vi "LilyPad_RB.vi"() -> ()   [LabVIEW 2012]
uses:
  <userlib>/BotSpeak/VIs/Direct/BotSpeak_Control.ctl
panel:
  in  "Bot Settings":T1
  out "List":string[](array[string])
  out "page":u8
  in  "Intro Help":bool
  in  "Previous":bool
  in  "Next":bool
  in  "Stop Button":bool
  in  "Pages":T2(tab)
  in  "Test Button":bool
  in  "Com Port":u16(ring)
  in  "Hardware":u16(ring) items=["Arduino Uno", "BeagleBone Serial", "BeagleBone", "Console Only", "EV3", "EvalRIO", "Launchpad", "PICAXE 80M", "Raspberry Pi", "Thymio"]
  out "firmware":dbl
  in  "Open":bool
  in  "Port":u8=13
  in  "State":enum16{"LO", "HI"}(ring)
  in  "Run":bool
  # "Getting Started\n\nThe goal of this book is to get you started in LabVIEW with the Lilypad - you will need 1 lilypad - please connect it up."
  # "Test BotSpeak\n\nThe next step is to test it out.  Choose your hardware and port (if you have not plugged your LilyPad in yet, plug it in and select Arduino Uno).  Push TEST to text the connection and see if you get Firmware 0.9 back."
  # "Test LilyPad\n\nPush the Run button - does the light go off?  Change it from LO to HI - and run it again.  What happens? Try changing the Port - from pin 13 to some other number.  This is called a LabVIEW diagram - it is where your program resides - this program is simple - it changes the state of pin 13.  Click on the Open button to open a slightly more complicated program."
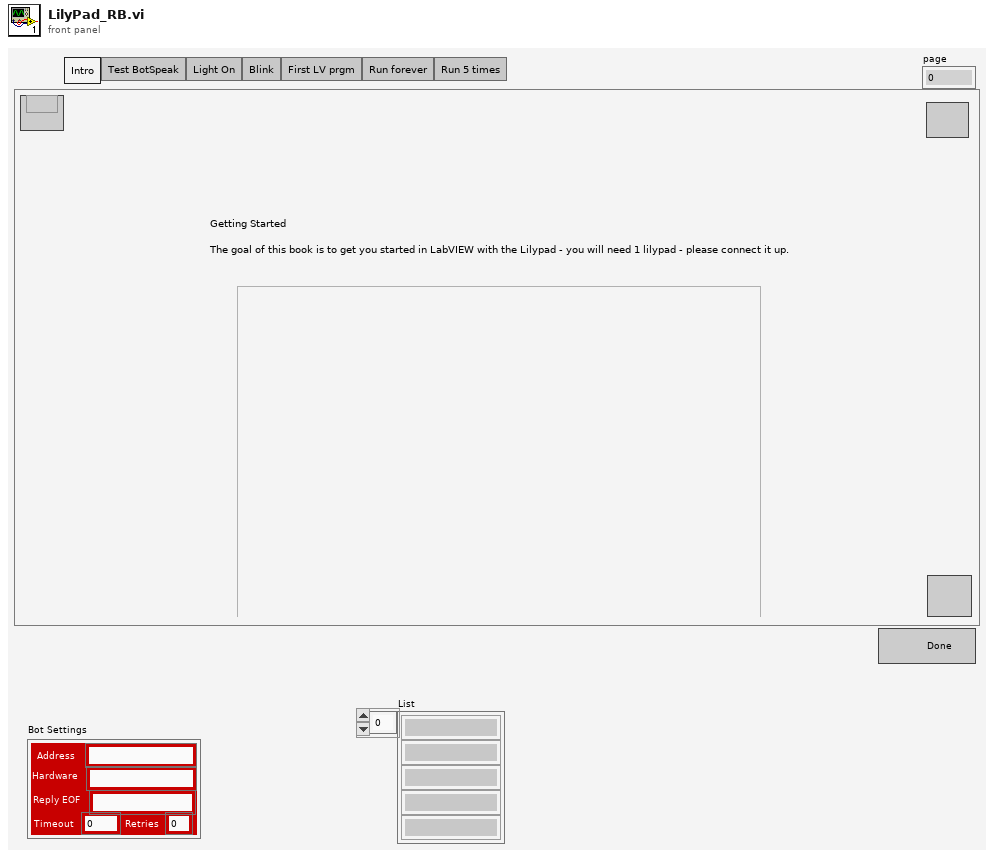
[diagram p1: front panel]
types:
  T1 = typedef "BotSpeak_Control.ctl" = cluster{"Address":string, "Reply EOF":string, "Hardware":string, "Retries":i8, "Timeout":i32}
  T2 = enum32{"Intro", "Test BotSpeak", "Light On", "Blink", "First LV prgm", "Run forever", "Run 5 times"}
  T3 = typedef "BotSpeak.HardwareSpecs.ctl" = cluster{"Hardware Name":string, "Hardware URL":string, "ComType":enum16{"Undefined", "Serial", "TCPIP", "Console", "EV3"}, "TCP Port":i32, "DefaultAddress":string, "Retries":i32, "Translate":enum16{"None", "Tiny", "URAPI"}, "MaxScriptSize":i32, "MaxVarNumber":i32, "StartupWait":i32, "Patience":i32, "Startup Patience":i32, "Hardware Help":string, "Com Protocol":string, "Translator":cluster{"BotSpeak CMD":string, "CMD out":string}[], "Init Code":string, "Variable Format":enum16{"INT", "FLOAT", "FIXED"}}
  T4 = enum16{"Undefined", "Serial", "TCPIP", "Console", "EV3"}
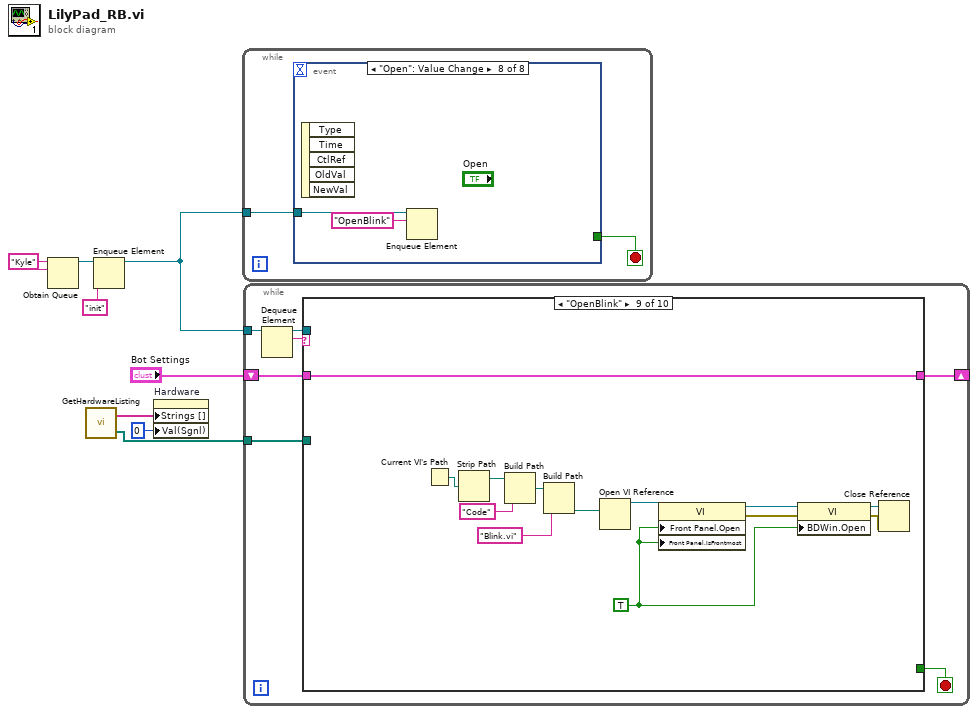
[diagram p0: block diagram]
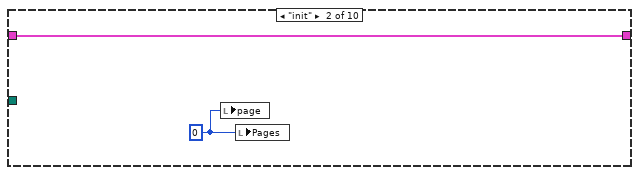
[diagram p3: hidden frame]
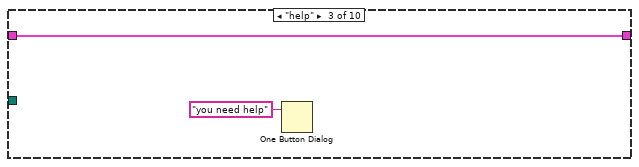
[diagram p4: hidden frame]
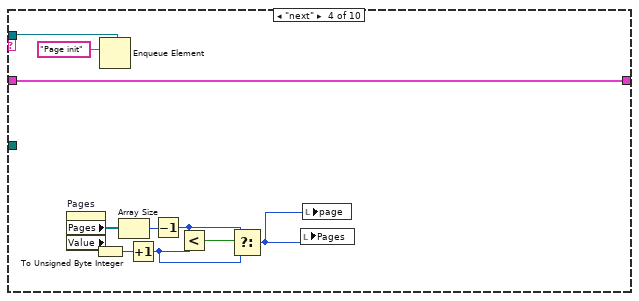
[diagram p5: hidden frame]
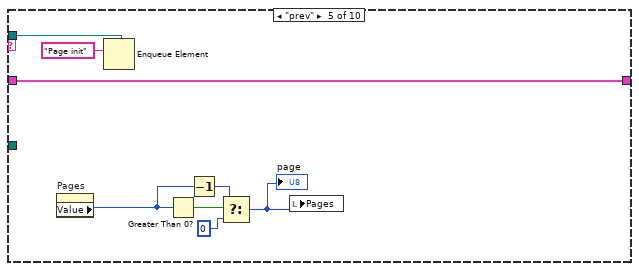
[diagram p6: hidden frame]
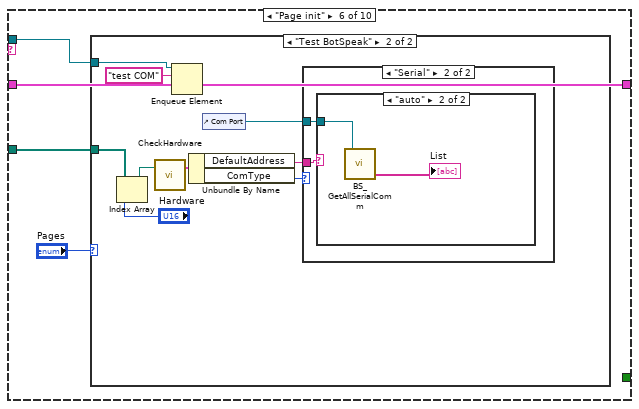
[diagram p7: hidden frame]
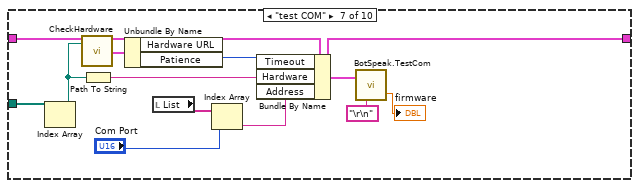
[diagram p11: hidden frame]
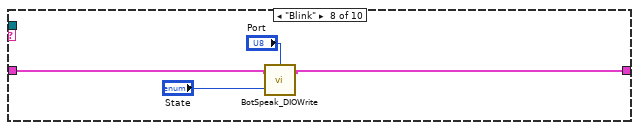
[diagram p12: hidden frame]
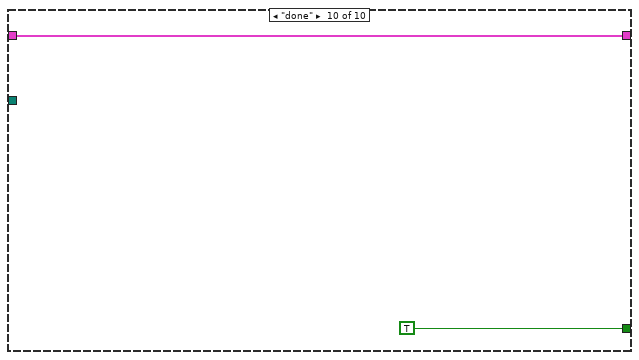
[diagram p13: hidden frame]
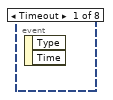
[diagram p14: hidden frame]
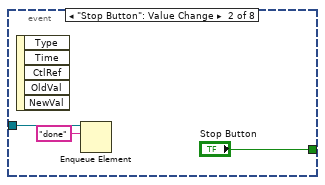
[diagram p15: hidden frame]
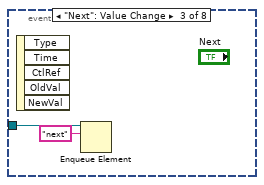
[diagram p16: hidden frame]
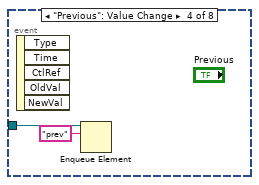
[diagram p17: hidden frame]
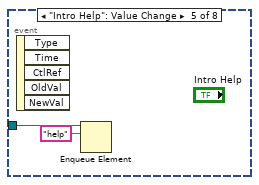
[diagram p18: hidden frame]
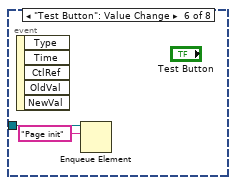
[diagram p19: hidden frame]
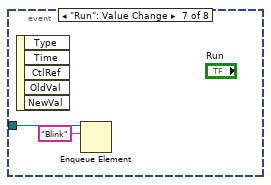
[diagram p20: hidden frame]
diagram:
  w7 = "Kyle" ("name (unnamed)")
  n1 = Obtain Queue(name (unnamed)=w7, element data type=w7) -> (queue out=w8:refnum<queue>)  [unwired: 3 in, 2 out]
  n2 = call <userlib>:"GetHardwareListing.vi"() -> ("Devices"=w2:path[], "Array"=w4:string[])  [unwired: 2 in]
  n3 = Enqueue Element(queue=w8, element="init") -> (queue out=w6:refnum<queue>)  [unwired: 2 in, 2 out]
  n4 = property on="Hardware" class="Ring (strict)"("Strings []"=w4, "Val(Sgnl)"=u16 0 ("Value (Signaling)")) -> ()  [unwired: 2 in, 2 out]
  n5 = while {
    tunnel: w6 -> [w9]
    stop <- w10 stop-if-true
    n6 = event shown="[7] \"Open\": Value Change" {
      selector: _ -> [_ _ _ _ _ _ _ _]
      dyn-events: _ -> [_ _ _ _ _ _ _ _]
      timeout: _ -> [_ _ _ _ _ _ _ _]
      tunnel: [_ "Stop Button" _ _ _ _ _ _] -> w10
      tunnel: w9 -> [_ w12 w15 w17 w19 w21 w23 w25]
      event Timeout {
        n7 = event-data() -> ()  [unwired: 1 in, 2 out]
      }
      event "Stop Button": Value Change {
        n8 = event-data() -> ()  [unwired: 1 in, 5 out]
        n9 = Enqueue Element(queue=w12, element="done") -> ()  [unwired: 2 in, 3 out]
      }
      event "Next": Value Change {
        n10 = event-data() -> ()  [unwired: 1 in, 5 out]
        n11 = Enqueue Element(queue=w15, element="next") -> ()  [unwired: 2 in, 3 out]
      }
      event "Previous": Value Change {
        n12 = event-data() -> ()  [unwired: 1 in, 5 out]
        n13 = Enqueue Element(queue=w17, element="prev") -> ()  [unwired: 2 in, 3 out]
      }
      event "Intro Help": Value Change {
        n14 = event-data() -> ()  [unwired: 1 in, 5 out]
        n15 = Enqueue Element(queue=w19, element="help") -> ()  [unwired: 2 in, 3 out]
      }
      event "Test Button": Value Change {
        n16 = event-data() -> ()  [unwired: 1 in, 5 out]
        n17 = Enqueue Element(queue=w21, element="Page init") -> ()  [unwired: 2 in, 3 out]
      }
      event "Run": Value Change {
        n18 = event-data() -> ()  [unwired: 1 in, 5 out]
        n19 = Enqueue Element(queue=w23, element="Blink") -> ()  [unwired: 2 in, 3 out]
      }
      event "Open": Value Change {
        n20 = event-data() -> ()  [unwired: 1 in, 5 out]
        n21 = Enqueue Element(queue=w25, element="OpenBlink") -> ()  [unwired: 2 in, 3 out]
      }
    }
  }
  n22 = while {
    tunnel: w6 -> [w32]
    tunnel: w2 -> [w28]
    shift-right: [w26] -> _
    shift-left: "Bot Settings" -> [w27]
    stop <- w30 stop-if-true
    n23 = Dequeue Element(queue=w32) -> (queue out=w29:refnum<queue>, element=w31:string)  [unwired: 2 in, 2 out]
    n24 = case shown="\"OpenBlink\"" w31 {
      tunnel: [_ _ _ _ _ _ _ _ _ TRUE] -> w30
      tunnel: w29 -> [_ _ _ w39 w50 w57 _ _ _ _]
      tunnel: w28 -> [_ _ _ _ _ w59 w78 _ _ _]
      tunnel: w27 -> [w33 w34 w36 w38 w49 w58 w76 w87 w102 w103]
      tunnel: [w33 w34 w36 w38 w49 w58 w74 w86 w102 w103] -> w26
      frame Default {
      }
      frame "init" {
        w35 = 0
        n25 = local write "page"(w35) -> ()
        n26 = local write "Pages"(w35) -> ()
      }
      frame "help" {
        n27 = One Button Dialog(message="you need help") -> ()  [unwired: 1 in, 1 out]
      }
      frame "next" {
        n28 = property on="Pages" class="TabCtl (strict)"() -> ("Pages"=w48:refnum<vi>[], "Value"=w45:T2)  [unwired: 2 in, 2 out]
        n29 = To Unsigned Byte Integer(number=w45) -> (unsigned 8bit integer=w42:u8)
        n30 = Enqueue Element(queue=w39, element="Page init") -> ()  [unwired: 2 in, 3 out]
        n31 = Array Size(array=w48) -> (size(s)=w46:i32)
        n32 = Increment(x=w42) -> (x+1=w44:u8)
        n33 = Decrement(x=w46) -> (x-1=w43:i32)
        n34 = Less?(x=w43, y=w44) -> (x < y?=w47:bool)
        n35 = Select(t=w43, s=w47, f=w44) -> (s? t:f=w41:i32)
        n36 = local write "Pages"(w41) -> ()
        n37 = local write "page"(w41) -> ()
      }
      frame "prev" {
        n38 = property on="Pages" class="TabCtl (strict)"() -> ("Value"=w53:T2)  [unwired: 2 in, 2 out]
        n39 = Enqueue Element(queue=w50, element="Page init") -> ()  [unwired: 2 in, 3 out]
        n40 = Greater Than 0?(x=w53) -> (x > 0?=w56:bool)
        n41 = Decrement(x=w53) -> (x-1=w52:T2)
        n42 = Select(t=w52, s=w56, f=0) -> (s? t:f=w54:u32)
        "page" <- w54
        n43 = local write "Pages"(w54) -> ()
      }
      frame "Page init" {
        n44 = case shown="\"Test BotSpeak\"" "Pages" {
          tunnel: w59 -> [_ w65]
          tunnel: w57 -> [_ w61]
          frame "Intro", Default {
          }
          frame "Test BotSpeak" {
            n45 = Index Array(array=w65, index="Hardware") -> (element=w66:path)
            n46 = call <userlib>:"CheckHardware.vi"("Hardware"=w66) -> ("HardwareSpecs"=w67:T3)  [unwired: 2 in]
            n47 = Enqueue Element(queue=w61, element="test COM") -> ()  [unwired: 2 in, 3 out]
            n48 = Unbundle By Name(w67) -> ("DefaultAddress"=w69:string, "ComType"=w68:T4)
            n49 = control-ref of="Com Port"() -> (w63:refnum<vi>)
            n50 = case shown="\"Serial\"" w68 {
              tunnel: w69 -> [_ w71]
              tunnel: w63 -> [_ w70]
              frame Default {
              }
              frame "Serial" {
                n51 = case shown="\"auto\"" w71 {
                  tunnel: w70 -> [_ w73]
                  frame Default {
                  }
                  frame "auto" {
                    n52 = call <userlib>:"BS_GetAllSerialComm.vi"("reference"=w73) -> ("List"=→"List":string[])  [unwired: 1 in, 2 out]
                  }
                }
              }
            }
          }
        }
      }
      frame "test COM" {
        n53 = Index Array(array=w78) -> (element=w81:path)  [unwired: 1 in]
        n54 = call <userlib>:"CheckHardware.vi"("Hardware"=w81) -> ("HardwareSpecs"=w80:T3)  [unwired: 2 in]
        n55 = Path To String(path=w81) -> (string=w83:string)
        n56 = Unbundle By Name(w80) -> ("Patience"=w82:i32)  [unwired: 1 out]
        n57 = local read "List"() -> (w79:string[])
        n58 = Index Array(array=w79, index="Com Port") -> (element=w75:string)
        n59 = Bundle By Name(cluster=w76, "Timeout"=w82, "Hardware"=w83, "Address"=w75) -> (w74:T1)
        n60 = call <userlib>:"BotSpeak.TestCom.vi"("Termination"="\r\n", "Bot Settings"=w74) -> ("firmware"=→"firmware":dbl)  [unwired: 1 out]
      }
      frame "Blink" {
        n61 = call <userlib>:"BotSpeak_DIOWrite.vi"("State"="State", "Bot Settings"=w87, "DIO Line"="Port") -> ("Bot Settings"=w86:T1)  [unwired: 1 out]
      }
      frame "OpenBlink" {
        w93 = TRUE ("Front Panel Window:Open")
        n62 = Current VI's Path() -> (path=w101:path)
        n63 = Strip Path(path=w101) -> (stripped path=w100:path)  [unwired: 1 out]
        n64 = Build Path(base path=w100, name or relative path="Code") -> (appended path=w98:path)
        n65 = Build Path(base path=w98, name or relative path="Blink.vi") -> (appended path=w96:path)
        n66 = Open VI Reference(vi path=w96) -> (vi reference=w92:refnum<vi>)  [unwired: 5 in, 1 out]
        n67 = property class="VI"(reference=w92, "Front Panel.Open"=w93, "Front Panel.IsFrontmost"=w93) -> (reference out=w95:refnum<vi>, error out=w94:errorcluster)  [unwired: 1 in]
        n68 = property class="VI"(reference=w95, error in=w94, "BDWin.Open"=w93) -> (reference out=w90:refnum<vi>, error out=w91:errorcluster)
        n69 = Close Reference(reference=w90, error in (no error)=w91) -> ()  [unwired: 1 out]
      }
      frame "done" {
      }
    }
  }
